vi "Choose Random Unvisited Neighbor.vi"(6 "Goal":T1, 8 "Width":i32, 9 "Height":i32, 10 "Position":T1, 11 "Visited":bool[][](array[boolean])) -> (0 "Valid?":bool, 3 "Random Unvisited Neighbor":T1)   [LabVIEW 2020, in "Maze.lvlib" / "MazeGen.lvclass"]
uses:
  MazeGen.lvclass
  Position.ctl
  Maze.lvlib
panel:
  out "Choices":i32
  out "Selected":i32
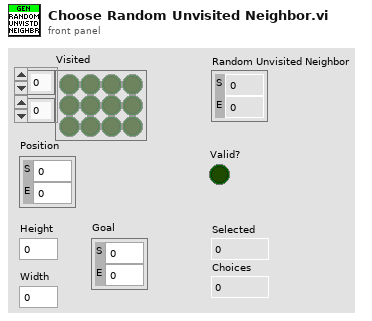
[diagram p1: front panel]
types:
  T1 = typedef "Maze.lvlib/Position.ctl" = cluster{"S":i32, "E":i32}
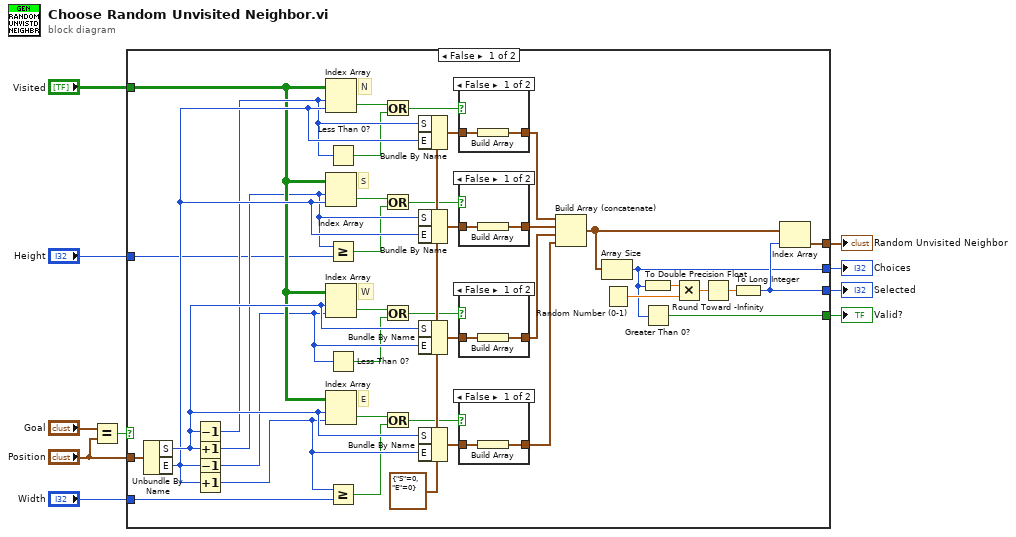
[diagram p0: block diagram]
diagram:
  n1 = Equal?(x="Goal", y="Position") -> (x = y?=w1:bool)
  n2 = case shown="False" w1 {
    tunnel: "Visited" -> [w40 _]
    tunnel: "Height" -> [w29 _]
    tunnel: "Width" -> [w27 _]
    tunnel: [w15 _] -> w7
    tunnel: [w14 _] -> w6
    tunnel: [w13 _] -> w5
    tunnel: [w12 _] -> w4
    tunnel: "Position" -> [w11 _]
    frame False {
      w48 = T1 {"S"=0, "E"=0} ("Position")
      # "S"
      # "W"
      # "E"
      # "N"
      n3 = Unbundle By Name(w11) -> ("S"=w50:i32, "E"=w49:i32)
      n4 = Decrement(x=w50) -> (x-1=w46:i32)
      n5 = Increment(x=w50) -> (x+1=w30:i32)
      n6 = Decrement(x=w49) -> (x-1=w32:i32)
      n7 = Increment(x=w49) -> (x+1=w26:i32)
      n8 = Index Array(array=w40, index (row)=w46, index (col)=w49) -> (element=w47:bool)
      n9 = Index Array(array=w40, index (row)=w30, index (col)=w49) -> (element=w41:bool)
      n10 = Index Array(array=w40, index (row)=w50, index (col)=w32) -> (element=w37:bool)
      n11 = Index Array(array=w40, index (row)=w50, index (col)=w26) -> (element=w34:bool)
      n12 = Less Than 0?(x=w46) -> (x < 0?=w45:bool)
      n13 = Greater Or Equal?(x=w30, y=w29) -> (x >= y?=w28:bool)
      n14 = Less Than 0?(x=w32) -> (x < 0?=w31:bool)
      n15 = Greater Or Equal?(x=w26, y=w27) -> (x >= y?=w25:bool)
      n16 = Or(x=w47, y=w45) -> (x .or. y?=w44:bool)
      n17 = Or(x=w41, y=w28) -> (x .or. y?=w42:bool)
      n18 = Or(x=w37, y=w31) -> (x .or. y?=w38:bool)
      n19 = Or(x=w34, y=w25) -> (x .or. y?=w35:bool)
      n20 = Bundle By Name(cluster=w48, "S"=w46, "E"=w49) -> (w43:T1)
      n21 = Bundle By Name(cluster=w48, "S"=w30, "E"=w49) -> (w39:T1)
      n22 = Bundle By Name(cluster=w48, "S"=w50, "E"=w32) -> (w36:T1)
      n23 = Bundle By Name(cluster=w48, "S"=w50, "E"=w26) -> (w33:T1)
      n24 = case shown="False" w44 {
        tunnel: w43 -> [w58 _]
        tunnel: [w57 _] -> w23
        frame False {
          n25 = Build Array(w58) -> (w57:T1[])
        }
        frame True {
        }
      }
      n26 = case shown="False" w42 {
        tunnel: w39 -> [w56 _]
        tunnel: [w55 _] -> w24
        frame False {
          n27 = Build Array(w56) -> (w55:T1[])
        }
        frame True {
        }
      }
      n28 = case shown="False" w38 {
        tunnel: w36 -> [w54 _]
        tunnel: [w53 _] -> w22
        frame False {
          n29 = Build Array(w54) -> (w53:T1[])
        }
        frame True {
        }
      }
      n30 = case shown="False" w35 {
        tunnel: w33 -> [w52 _]
        tunnel: [w51 _] -> w21
        frame False {
          n31 = Build Array(w52) -> (w51:T1[])
        }
        frame True {
        }
      }
      n32 = Build Array (concatenate)(w23, w24, w22, w21) -> (w16:T1[])
      n33 = Array Size(array=w16) -> (size(s)=w13:i32)
      n34 = Random Number (0-1)() -> (number: 0 to 1=w19:dbl)
      n35 = To Double Precision Float(number=w13) -> (double precision float=w20:dbl)
      n36 = Greater Than 0?(x=w13) -> (x > 0?=w12:bool)
      n37 = Multiply(x=w20, y=w19) -> (x*y=w18:dbl)
      n38 = Round Toward -Infinity(1:w18) -> (0:w17:dbl)
      n39 = To Long Integer(number=w17) -> (32bit integer=w15:i32)
      n40 = Index Array(array=w16, index=w15) -> (element=w14:T1)
    }
    frame True {
    }
  }
  "Selected" <- w7
  "Choices" <- w5
  "Random Unvisited Neighbor" <- w6
  "Valid?" <- w4
